vi "컴퓨터 ProcessID.vi"() -> ()   [LabVIEW 2014]
uses:
  Windows/System32/kernel32.dll
  winmm.dll
panel:
  out "Success?":bool
  in  "경로":path
  out "ComputerName":string
  out "Current ProcessID":i32
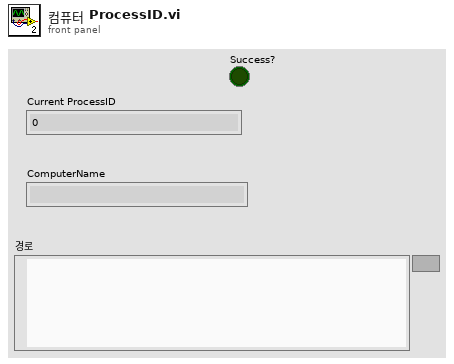
[diagram p1: front panel]
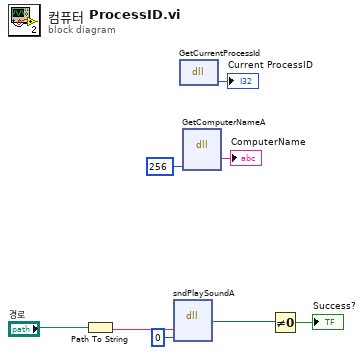
[diagram p0: block diagram]
diagram:
  n1 = Path To String(path="경로") -> (string=w4:string)
  n2 = dll-call lib="winmm.dll" fn="sndPlaySoundA"("SoundFile"=w4, "options"=u32 0) -> ("반환 타입"=w2:i32)  [unwired: 5 in, 2 out]
  n3 = dll-call lib="C:/Windows/System32/kernel32.dll" fn="GetCurrentProcessId"() -> ("반환 타입"=→"Current ProcessID":i32)  [unwired: 3 in, 2 out]
  n4 = dll-call lib="C:/Windows/System32/kernel32.dll" fn="GetComputerNameA"("ln"=u32 256) -> ("ComputerName"=→"ComputerName":string)  [unwired: 6 in, 2 out]
  n5 = Not Equal To 0?(x=w2) -> (x != 0?=→"Success?":bool)
